vi "(SubVI) Stop a Sine Wave Generation.vi"(4 "error in (no error)":errorcluster, 6 "Axis  (Enum)":enum16{"x", "y", "z"}(ring)) -> (0 "error out":errorcluster)   [LabVIEW 2014]
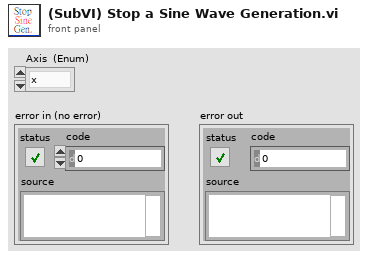
[diagram p1: front panel]
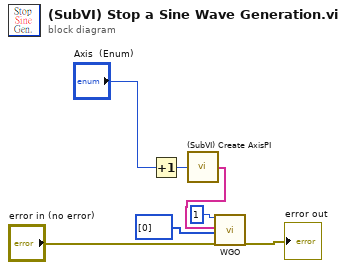
[diagram p0: block diagram]
diagram:
  n1 = Increment(x="Axis  (Enum)") -> (x+1=w6:enum16{"x", "y", "z"})
  n2 = call "(SubVI) Create AxisPI.vi"("axis"=w6) -> ("Axis String Array"=w7:string[])  [unwired: 2 in, 2 out]
  n3 = call "WGO.vi"("System no."=1, "Affected axes"=w7, "WGO Parameter"=i32[] [0], "error in"="error in (no error)") -> ("error out"=→"error out":errorcluster)  [unwired: 15 out]
